vi "RecordingParameterAddress.vi"(8 "error in (no error)":errorcluster, 11 "StepMotor in":refnum<class "StepMotor.lvclass">) -> (0 "error out":errorcluster, 3 "StepMotor out":refnum<class "StepMotor.lvclass">)   [LabVIEW 2010, in "StepMotor.lvclass"]
doc: "Запись парметра по адресу в СПШ."
uses:
  StepMotor.lvclass
  StepMotor.lvclass/StepMotor.ctl
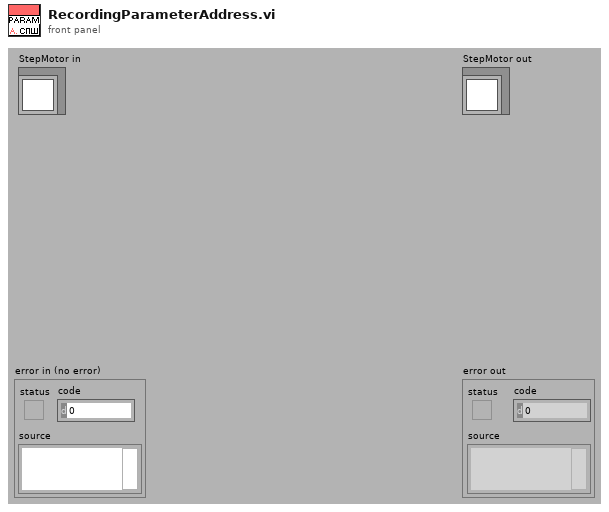
[diagram p1: front panel]
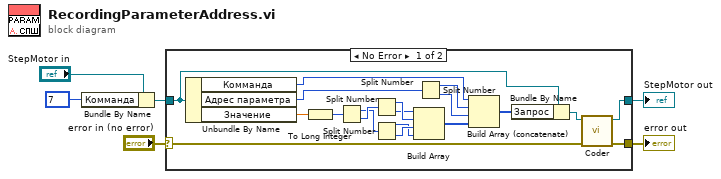
[diagram p0: block diagram]
diagram:
  n1 = Bundle By Name(cluster="StepMotor in", "Комманда"=u8 7 ("Numeric")) -> (w4:refnum<class "StepMotor.lvclass">)
  n2 = case shown="No Error" "error in (no error)" {
    selector: "error in (no error)" -> [w19 w27]
    tunnel: [w20 w26] -> w2
    tunnel: w4 -> [w23 w26]
    tunnel: [w18 w27] -> w6
    frame No Error {
      n3 = Unbundle By Name(w23) -> ("Комманда"=w9:u8, "Адрес параметра"=w25:u16, "Значение"=w8:dbl)
      n4 = To Long Integer(number=w8) -> (32bit integer=w7:i32)
      n5 = Split Number(x=w7) -> (hi(x)=w16:u16, lo(x)=w17:u16)
      n6 = Split Number(x=w17) -> (hi(x)=w13:u8, lo(x)=w12:u8)
      n7 = Split Number(x=w16) -> (hi(x)=w14:u8, lo(x)=w15:u8)
      n8 = Build Array(w12, w13, w15, w14) -> (w24:u8[])
      n9 = Split Number(x=w25) -> (hi(x)=w11:u8, lo(x)=w10:u8)
      n10 = Build Array (concatenate)(w9, w11, w10, w24) -> (w22:u8[])
      n11 = Bundle By Name(cluster=w23, "Запрос"=w22) -> (w21:refnum<class "StepMotor.lvclass">)
      n12 = call "Coder.vi"("error in (no error)"=w19, "StepMotor in"=w21) -> ("error out"=w18:errorcluster, "StepMotor out"=w20:refnum<class "StepMotor.lvclass">)  [unwired: 8 in]
    }
    frame Error {
    }
  }
  "error out" <- w6
  "StepMotor out" <- w2
